vi "LoadCombinations.vi"() -> ()   [LabVIEW 2016]
panel:
  in  "LoadCombinations":i32[][](array[numeric])
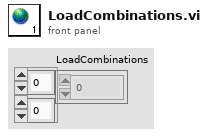
[diagram p1: front panel]
diagram:
